vi "Tridiagonal LU Decomposition (DBL).vi"(9 "Super Diagonal":dbl[](array[numeric]), 10 "Diagonal":dbl[](array[numeric]), 11 "Sub Diagonal":dbl[](array[numeric])) -> (0 "error":i32, 1 "Pivot":i32[](array[numeric]), 2 "U":T1, 3 "L":dbl[](array[numeric]))   [LabVIEW 2020, in "NI_AALPro.lvlib"]
uses:
  <vilib>/Analysis/NI_AALPro.lvlib
  <resource>/lvanlys.dll
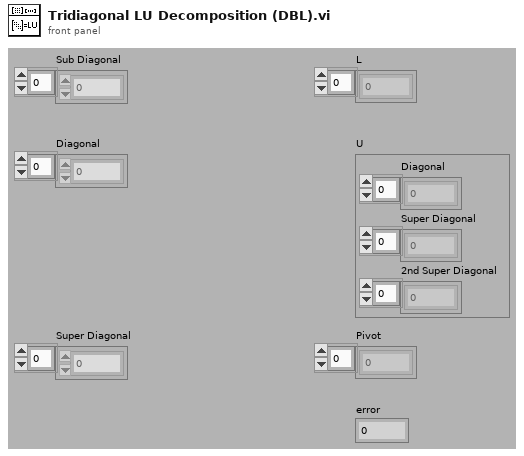
[diagram p1: front panel]
types:
  T1 = cluster{"Diagonal":dbl[], "Super Diagonal":dbl[], "2nd Super Diagonal":dbl[]}
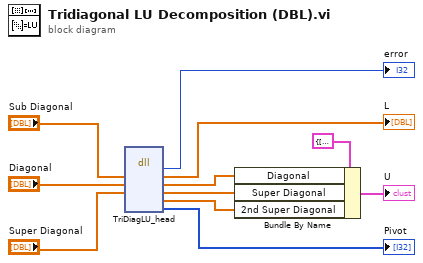
[diagram p0: block diagram]
diagram:
  n1 = dll-call lib="e:/builds/penguin/labview/branches/2020/dev/dist/resource/lvanlys.*" fn="TriDiagLU_head" ("CBLAS.dll:MtrxxVectH")("SubDiag"="Sub Diagonal", "Diag"="Diagonal", "SuperDiag"="Super Diagonal") -> ("error"=→"error":i32, "SubDiag"=→"L":dbl[], "Diag"=w8:dbl[], "SuperDiag"=w7:dbl[], "SuperDiag2"=w6:dbl[], "PVT"=→"Pivot":i32[])  [unwired: 3 in, 4 out]
  n2 = Bundle By Name(cluster=T1 {"Diagonal"=[], "Super Diagonal"=[], "2nd Super Diagonal"=[]} ("U"), "Diagonal"=w8, "Super Diagonal"=w7, "2nd Super Diagonal"=w6) -> (→"U":T1)
